vi "Update Position.vi"(8 "Direction":T1, 9 "Action":T2, 10 "Replicated in":refnum<class "Border.lvclass">, 11 "64 in":refnum<class "Border.lvclass">) -> (2 "Replicated out":refnum<class "Border.lvclass">, 3 "64 out":refnum<class "Border.lvclass">)   [LabVIEW 2015, in "Border.lvclass"]
uses:
  Border.lvclass
  Type Defs/Action Enum.ctl
  Type Defs/Direction Enum.ctl
  Border.lvclass/Border.ctl
  Square/Board Size.vi
  SubVIs/Read-Only Globals.vi
  SubVIs/Globals (private).vi
  Common/Common.lvlib
  Type Defs/SB Type Defs.lvlib
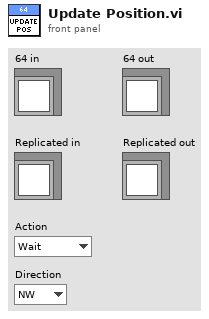
[diagram p1: front panel]
types:
  T1 = typedef "SB Type Defs.lvlib/Direction Enum.ctl" = enum16{"NW", "N", "NE", "E", "SE", "S", "SW", "W"}
  T2 = typedef "SB Type Defs.lvlib/Action Enum.ctl" = enum16{"Wait", "Move", "Attack", "Replicate"}
  T3 = typedef "Common.lvlib/Position.ctl" = cluster{"Column":i32, "Row":i32}
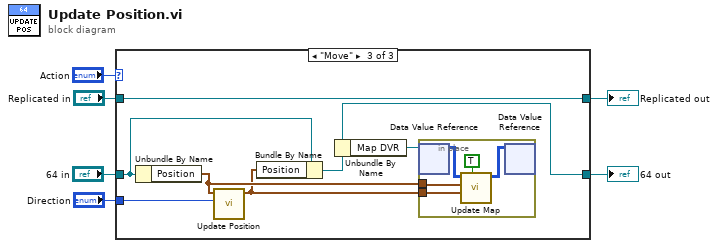
[diagram p0: block diagram]
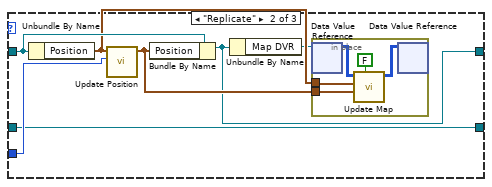
[diagram p3: hidden frame]
diagram:
  n1 = case shown="\"Move\"" "Action" {
    tunnel: "Replicated in" -> [w7 w14 w25]
    tunnel: "Direction" -> [_ w15 w27]
    tunnel: [w7 w10 w25] -> w3
    tunnel: "64 in" -> [w8 w13 w26]
    tunnel: [w8 w13 w22] -> w1
    frame Default {
    }
    frame "Replicate" {
      n2 = Unbundle By Name(w14) -> ("Position"=w12:T3)
      n3 = call "Update Position.vi"("Direction"=w15, "Position in"=w12) -> ("Position out"=w11:T3)  [unwired: 9 in]
      n4 = Bundle By Name(cluster=w14, "Position"=w11) -> (w10:refnum<class "Border.lvclass">)
      n5 = Unbundle By Name(w10) -> ("Map DVR"=w9:refnum<data-value>)
      n6 = in-place {
        in-place-border: w12 -> [w20]
        in-place-border: w11 -> [w19]
        n7 = in-place-dvr #1(w9) -> (w17:i32[][])  [unwired: 1 out]
        n8 = call "Update Map.vi"("Moved?"=FALSE, "New Position"=w19, "Old Position"=w20, "Map in"=w17) -> ("Map"=w16:i32[][])  [unwired: 7 in]
        n9 = in-place-dvr #1(w16) -> ()  [unwired: 2 out]
      }
    }
    frame "Move" {
      n10 = Unbundle By Name(w26) -> ("Position"=w24:T3)
      n11 = call "Update Position.vi"("Direction"=w27, "Position in"=w24) -> ("Position out"=w23:T3)  [unwired: 9 in]
      n12 = Bundle By Name(cluster=w26, "Position"=w23) -> (w22:refnum<class "Border.lvclass">)
      n13 = Unbundle By Name(w22) -> ("Map DVR"=w21:refnum<data-value>)
      n14 = in-place {
        in-place-border: w24 -> [w32]
        in-place-border: w23 -> [w31]
        n15 = in-place-dvr #2(w21) -> (w29:i32[][])  [unwired: 1 out]
        n16 = call "Update Map.vi"("Moved?"=TRUE, "New Position"=w31, "Old Position"=w32, "Map in"=w29) -> ("Map"=w28:i32[][])  [unwired: 7 in]
        n17 = in-place-dvr #2(w28) -> ()  [unwired: 2 out]
      }
    }
  }
  "64 out" <- w1
  "Replicated out" <- w3
